vi "Calculate X Y Waveform Voltage Out Whole Image.vi"(7 "Raster Scan Direction":T1, 8 "Y Flyback":dbl[][](graph), 9 "Y Waveform":dbl[](graph), 10 "X Flyback":dbl[][](graph), 11 "X Waveform":dbl[](graph)) -> (1 "Y Waveform Out":dbl[](graph), 3 "X Waveform Out":dbl[](graph), 4 "Digital Line Acq":bool[](array[boolean]), 5 "XY Waveform Out":dbl[][](graph))   [LabVIEW 2018]
uses:
  Controls/Scan Direction.ctl
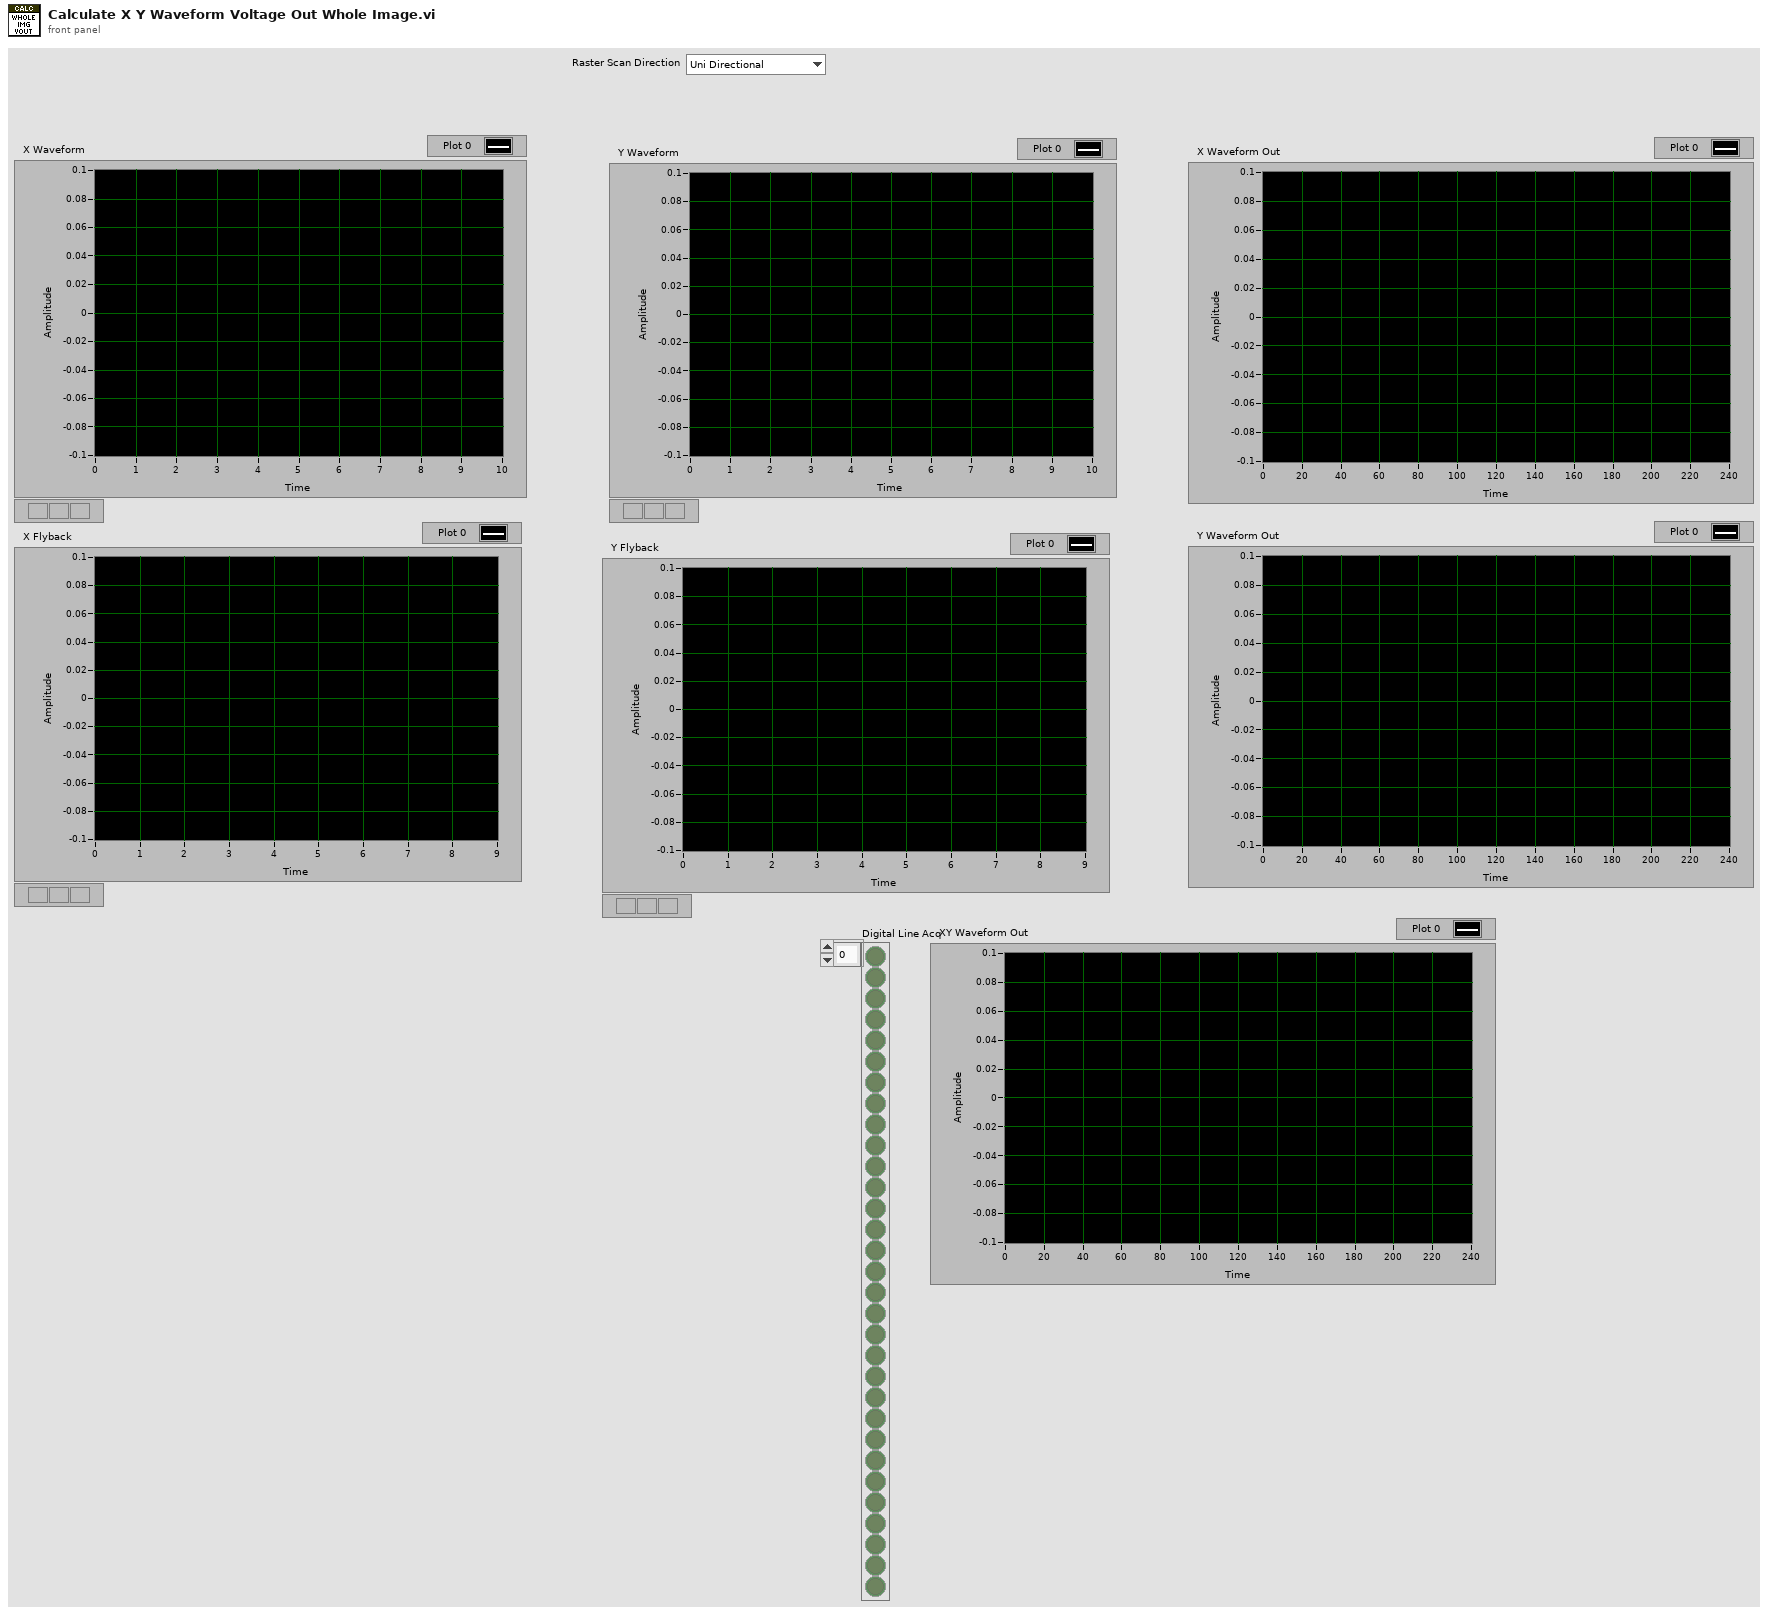
[diagram p1: front panel]
types:
  T1 = typedef "Scan Direction.ctl" = enum16{"Uni Directional", "Bi Directional", "None"}
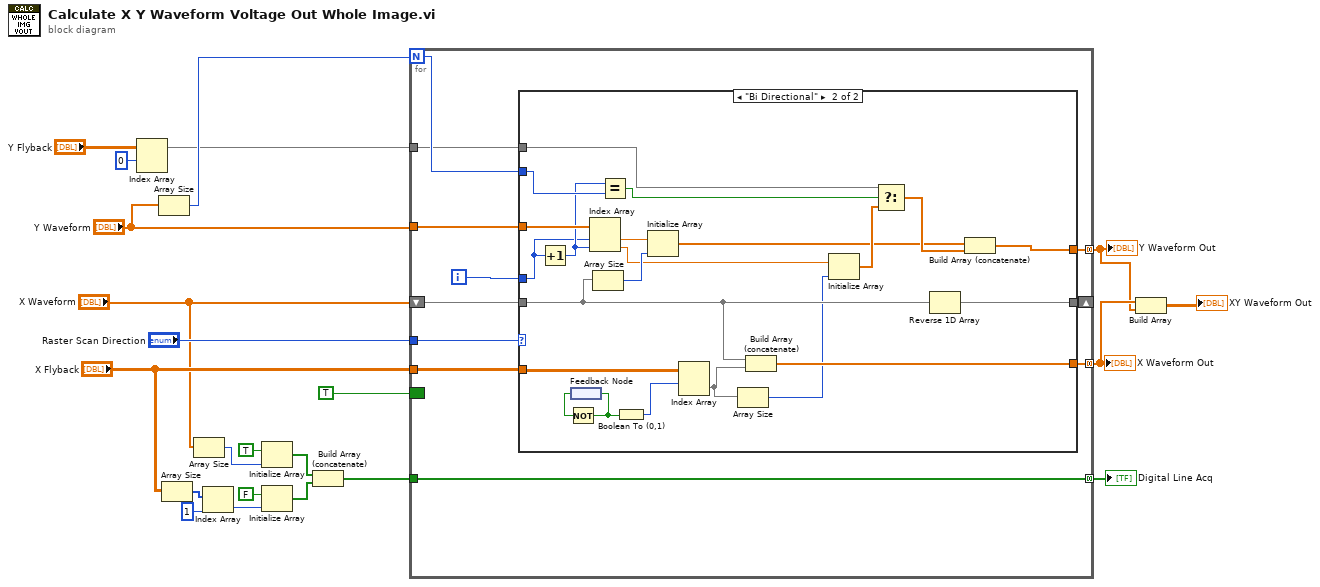
[diagram p0: block diagram]
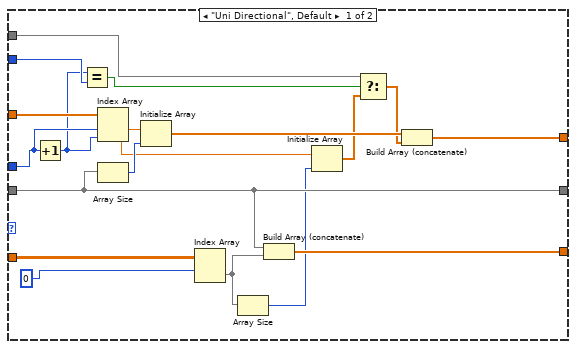
[diagram p2: hidden frame]
diagram:
  n1 = Index Array(array="Y Flyback", index (row)=0) -> (element=w18:dbl[])  [unwired: 1 in]
  n2 = Array Size(array="Y Waveform") -> (size(s)=w20:i32)
  n3 = Array Size(array="X Flyback") -> (size(s)=w11:i32[])
  n4 = Array Size(array="X Waveform") -> (size(s)=w6:i32)
  n5 = Index Array(array=w11, index=1) -> (element=w10:i32)
  n6 = Initialize Array(TRUE, w6) -> (w5:bool[])
  n7 = Initialize Array(FALSE, w10) -> (w4:bool[])
  n8 = Build Array (concatenate)(w5, w4) -> (w3:bool[])
  n9 = for {
    N: w20 -> [w25]
    shift-right: [w33] -> _
    shift-left: "X Waveform" -> [w32]
    tunnel: "Raster Scan Direction" -> [w31]
    tunnel: "Y Waveform" -> [w27]
    tunnel: "X Flyback" -> [w30]
    tunnel: [w28] -> w16 mode=concatenating
    tunnel: [w26] -> w15 mode=concatenating
    tunnel: w18 -> [w24]
    border: TRUE -> [_]
    tunnel: w3 -> [w23]
    tunnel: [w23] -> w2 mode=concatenating
    i -> [w29]
    n10 = case shown="\"Bi Directional\"" w31 {
      tunnel: [w46 w74] -> w33
      tunnel: w32 -> [w46 w64]
      tunnel: w30 -> [w52 w73]
      tunnel: w29 -> [w40 w66]
      tunnel: [w50 w72] -> w28
      tunnel: w27 -> [w49 w68]
      tunnel: [w41 w57] -> w26
      tunnel: w25 -> [w39 w69]
      tunnel: w24 -> [w35 w70]
      frame "Uni Directional", Default {
        n11 = Increment(x=w40) -> (x+1=w34:i32)
        n12 = Equal?(x=w34, y=w39) -> (x = y?=w38:bool)
        n13 = Index Array(array=w49, index #1=w40, index #2=w34) -> (element #1=w48:dbl, element #2=w45:dbl)
        n14 = Array Size(array=w46) -> (size(s)=w47:i32)
        n15 = Initialize Array(w48, w47) -> (w42:dbl[])
        n16 = Index Array(array=w52, index (row)=0 ("disabled index (col)")) -> (element=w44:dbl[])  [unwired: 1 in]
        n17 = Array Size(array=w44) -> (size(s)=w43:i32)
        n18 = Build Array (concatenate)(w46, w44) -> (w50:dbl[])
        n19 = Initialize Array(w45, w43) -> (w36:dbl[])
        n20 = Select(t=w35, s=w38, f=w36) -> (s? t:f=w37:dbl[])
        n21 = Build Array (concatenate)(w42, w37) -> (w41:dbl[])
      }
      frame "Bi Directional" {
        n22 = Increment(x=w66) -> (x+1=w67:i32)
        n23 = feedback #1() -> (w55:bool)
        n24 = Not(x=w55) -> (.not. x?=w54:bool)
        n25 = feedback-in #1(w54) -> ()
        n26 = Index Array(array=w68, index #1=w66, index #2=w67) -> (element #1=w65:dbl, element #2=w62:dbl)
        n27 = Array Size(array=w64) -> (size(s)=w63:i32)
        n28 = Equal?(x=w67, y=w69) -> (x = y?=w71:bool)
        n29 = Boolean To (0,1)(Boolean=w54) -> (0, 1=w53:i16)
        n30 = Initialize Array(w65, w63) -> (w56:dbl[])
        n31 = Index Array(array=w73, index (row)=w53) -> (element=w60:dbl[])  [unwired: 1 in]
        n32 = Array Size(array=w60) -> (size(s)=w59:i32)
        n33 = Build Array (concatenate)(w64, w60) -> (w72:dbl[])
        n34 = Initialize Array(w62, w59) -> (w61:dbl[])
        n35 = Select(t=w70, s=w71, f=w61) -> (s? t:f=w58:dbl[])
        n36 = Reverse 1D Array(array=w64) -> (reversed array=w74:dbl[])
        n37 = Build Array (concatenate)(w56, w58) -> (w57:dbl[])
      }
    }
  }
  "X Waveform Out" <- w16
  "Y Waveform Out" <- w15
  "Digital Line Acq" <- w2
  n38 = Build Array(w16, w15) -> (→"XY Waveform Out":dbl[][])
